vi "Tool specific Variable List.vi"(11 "error in (no error)":errorcluster) -> (15 "error out":errorcluster)   [LabVIEW 2011]
uses:
  emi Lib/Basic/0 - General/App/emi_Application Folder.vi
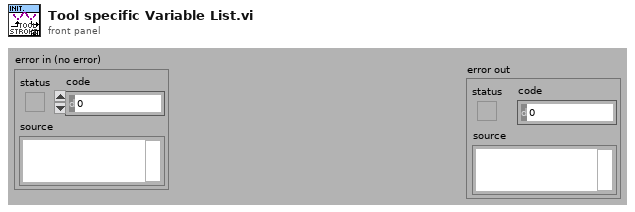
[diagram p1: front panel]
types:
  T1 = typedef "Fixed Analog Channel Definition.ctl" = cluster{"ID":u16, "Name":string, "Quantity":T2, "Unit":string, "Maximum upd":T3, "Comment":string, "Help file Name":string, "Help file Section ":string, "Category":T4, "User adjustable Scaling":bool, "Default Scaling":T5, "Default Unit":i32, "Classification":T6}
  T2 = typedef "Quantity enum.ctl" = enum16{"NA", "Acceleration", "Angle", "Current", "Force", "Distance", "Pressure", "Resistance", "Rotational Speed", "Speed", "Temperature", "Tension", "Torque", "Voltage", "Weight"}
  T3 = typedef "Update frequensies.ctl" = enum16{"2 Hz", "1 Hz", "0.1 Hz"}
  T4 = typedef "Channel catagory Enum.ctl" = enum16{"No Category", "Power", "Temperature", "Pressure"}
  T5 = typedef "Scaling.ctl" = cluster{"Gain":dbl, "Offset":dbl}
  T6 = typedef "Channel Classification Enum.ctl" = enum16{"Basic", "Advanced", "Expert", "Unused"}
  T7 = typedef "Fixed Digital Channel Definition.ctl" = cluster{"ID":u16, "Name":string, "NA Text":string, "Off Text":string, "On Text":string, "Maximum upd":T3, "Comment":string, "Help file Name":string, "Help file Section ":string, "Catagory":T4, "In use":bool}
  T8 = typedef "User Setting DigitalChannel.ctl" = cluster{"Responses":cluster{"Technical Error (NA)":T9, "OFF / FALSE":T11, "ON / TRUE":T11}}
  T9 = typedef "Alarm Responce.ctl" = cluster{"Action":T10, "Alarm":bool}
  T10 = typedef "Action List.ctl" = enum16{"No Action", "Stop Motor", "Turn Off HV"}
  T11 = typedef "Alarm Responce dig.ctl" = cluster{"Action":T10, "Alarm":bool, "Exclamation":bool}
  T12 = typedef "User Setting Analog Channel Bg.ctl" = cluster{"Scaling":T5, "Limits and responces":T13, "Allow Graph selection by user":bool, "Unit":u16}
  T13 = typedef "Alarm Setup Analog.ctl" = cluster{"Technical Error(NA)":T9, "LL":T9, "L":T9, "H":T9, "HH":T9, "Limits":T14}
  T14 = typedef "Limits.ctl" = cluster{"LL":dbl, "L":dbl, "H":dbl, "HH":dbl}
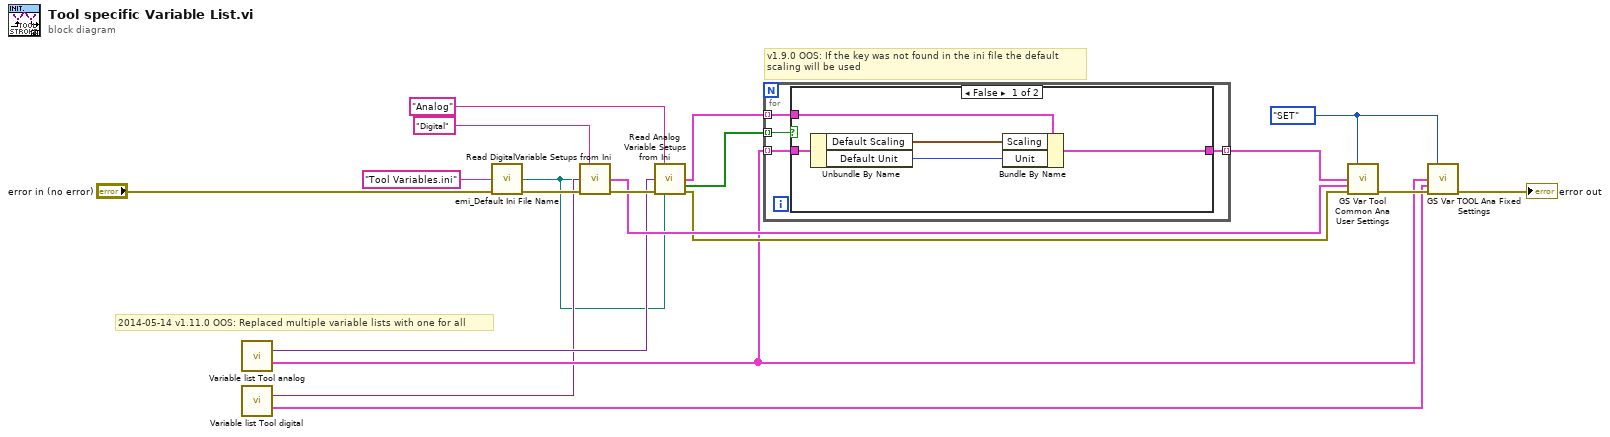
[diagram p0: block diagram]
diagram:
  w16 = enum16{"GET", "SET"}."SET" ("Action(GET)")
  # "2014-05-14 v1.11.0 OOS: Replaced multiple variable lists with one for all"
  # "v1.9.0 OOS: If the key was not found in the ini file the default\nscaling will be used"
  n1 = call "Variable list Tool analog.vi"() -> ("Variant"=w8:variant, "Array"=w7:T1[])  [unwired: 14 in]
  n2 = call "Variable list Tool digital.vi"() -> ("Variant"=w4:variant, "Array"=w3:T7[])  [unwired: 14 in]
  n3 = call "emi_Default Ini File Name.vi"("Name"="Tool Variables.ini" ("name or relative path"), "error in (no error)"="error in (no error)") -> ("Path"=w2:path, "error out"=w6:errorcluster)  [unwired: 12 in]
  n4 = call "Read DigitalVariable Setups from Ini.vi"("error in (no error)"=w6, "Path"=w2, "Enum with Variable List"=w4, "Section(\"Default\")"="Digital" ("Section(\"Default\")")) -> ("error out"=w15:errorcluster, "Digitale User settigns"=w13:T8[])  [unwired: 10 in]
  n5 = call "Read Analog Variable Setups from Ini.vi"("error in (no error)"=w15, "Path"=w2, "Enum with Variable List"=w8, "Section(\"Default\")"="Analog" ("Section(\"Default\")")) -> ("error out"=w9:errorcluster, "Found out"=w11:bool[], "Analog User settigns"=w12:T12[])  [unwired: 9 in]
  n6 = for {
    tunnel: w12 -> [w22] mode=indexing
    tunnel: w11 -> [w23] mode=indexing
    tunnel: w7 -> [w21] mode=indexing
    tunnel: [w20] -> w10 mode=indexing
    n7 = case shown="False" w23 {
      tunnel: w22 -> [w28 w29]
      tunnel: w21 -> [w27 _]
      tunnel: [w24 w29] -> w20
      frame False {
        n8 = Unbundle By Name(w27) -> ("Default Scaling"=w26:T5, "Default Unit"=w25:i32)
        n9 = Bundle By Name(cluster=w28, "Scaling"=w26, "Unit"=w25) -> (w24:T12)
      }
      frame True {
      }
    }
  }
  n10 = call "GS Var Tool Common Ana User Settings.vi"("Action(GET)"=w16, "Tool analog var User settigns in"=w10, "Tool digital var User settigns in"=w13, "error in (no error)"=w9) -> ("error out"=w18:errorcluster)  [unwired: 9 in, 2 out]
  n11 = call "GS Var TOOL Ana Fixed Settings.vi"("Action(GET)"=w16, "Tool Analog Var Fixed in"=w7, "Tool Digital Var Fixed in"=w3, "error in (no error)"=w18) -> ("error out"=→"error out":errorcluster)  [unwired: 9 in, 2 out]
